vi "Initialize Sessions - 1Sess.vi"(6 "initialize and close session behavior":T1, 7 "serial configuration":T2, 8 "error in":errorcluster, 9 "reset":bool, 11 "session reservation in":refnum<class "Session Reservation.lvclass">) -> (0 "error out":errorcluster, 1 "channel list":string, 2 "session":refnum<visa-resource-name>, 3 "session reservation out":refnum<class "Session Reservation.lvclass">)   [LabVIEW 2020, in "Keysight 34401A DMM Instrument.lvlib"]
doc: "Create the 34401 driver session from the <b>session reservation in</b>. Returns an error if more than one 34401 session has been reserved. Use \"Create Session - NSess.vi\" for multiple sessions."
uses:
  Keysight 34401A DMM Instrument.lvlib
  <vilib>/MeasurementLink/MeasurementLink Session Management V1/Session Reservation/Session Reservation.lvclass
  <vilib>/MeasurementLink/MeasurementLink Session Management V1/Session Reservation/Initialize and Close Session Behavior.ctl
  52dcdb1e-5454-43fd-959d-10a398c05520.vi
  Session Factory/Session Factory.lvclass
  C:/Program Files/National Instruments/LabVIEW 2020/vi.lib/MeasurementLink/MeasurementLink Instrument/ISession Factory/ISession Factory.lvclass
  <vilib>/MeasurementLink/MeasurementLink Session Management V1/Session Reservation/Initialize Sessions with Retry.vi
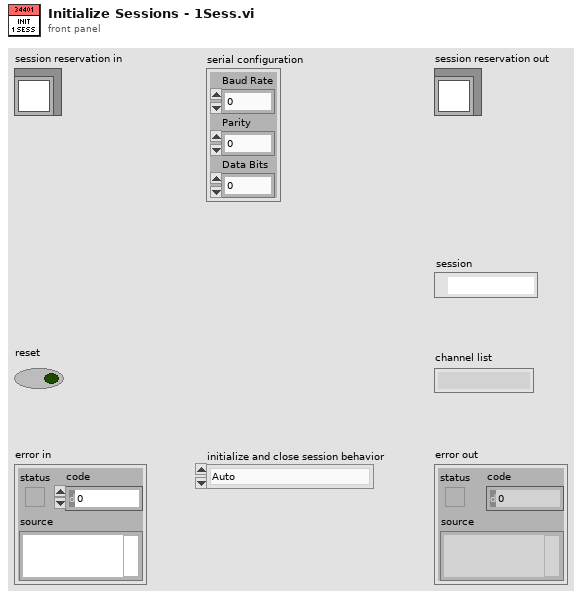
[diagram p1: front panel]
types:
  T1 = typedef "MeasurementLink Session Management V1.lvlib/Session Reservation.lvclass/Initialize and Close Session Behavior.ctl" = enum16{"Auto", "Initialize and Close", "Attach and Detach", "Initialize and Detach", "Attach and Close"}
  T2 = cluster{"Baud Rate":u32, "Parity":u16, "Data Bits":u16}
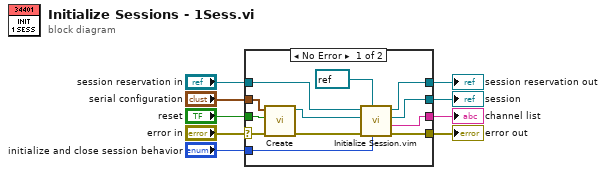
[diagram p0: block diagram]
diagram:
  n1 = case shown="No Error" "error in" {
    selector: "error in" -> [w20 w23]
    tunnel: [w18 w23] -> w8
    tunnel: [w21 w22] -> w6
    tunnel: "session reservation in" -> [w14 w22]
    tunnel: "reset" -> [w19 _]
    tunnel: [w17 _] -> w4
    tunnel: [w16 _] -> w2
    tunnel: "serial configuration" -> [w12 _]
    tunnel: "initialize and close session behavior" -> [w10 _]
    frame No Error {
      n2 = call "Create.vi"("error in"=w20, "reset"=w19, "serial configuration"=w12) -> ("error out"=w13:errorcluster, "session factory out"=w15:refnum<class "Session Factory.lvclass">)  [unwired: 7 in]
      n3 = call "Initialize Session.vim"("initialize and close session behavior"=w10, "session type"=refnum<visa-resource-name> refnum ("session"), "error in"=w13, "session factory"=w15, "session reservation in"=w14) -> ("error out"=w18:errorcluster, "channel list"=w17:string, "session"=w16:refnum<visa-resource-name>, "session reservation out"=w21:refnum<class "Session Reservation.lvclass">)  [unwired: 3 in]
    }
    frame Error {
    }
  }
  "error out" <- w8
  "session reservation out" <- w6
  "channel list" <- w4
  "session" <- w2
